vi "Turret_Execute.vi"() -> ()   [LabVIEW 2019]
uses:
  Turret_States.ctl
  <vilib>/Rock Robotics/WPI/ThirdParty/REV Robotics/SPARK MAX/Typedef/Spark MAX Control Type.ctl
  Globals/Turret_Globals.vi
  Globals/Sensor_Values.vi
panel:
  out "Waveform Chart":cluster{"Goal Wheel Position":dbl, dbl}(graph)
  in  "Kp_Degrees":dbl=0.07
  in  "Kd Aim":dbl=0.001
  in  "Ki Aim":dbl=1e-05
  in  "upper_limit(degrees)":dbl=135.0
  in  "lower_limit(degrees)":dbl=-83.0
  out "Turret_Spin_Speed":dbl
  in  "Kp Aim":dbl=0.06
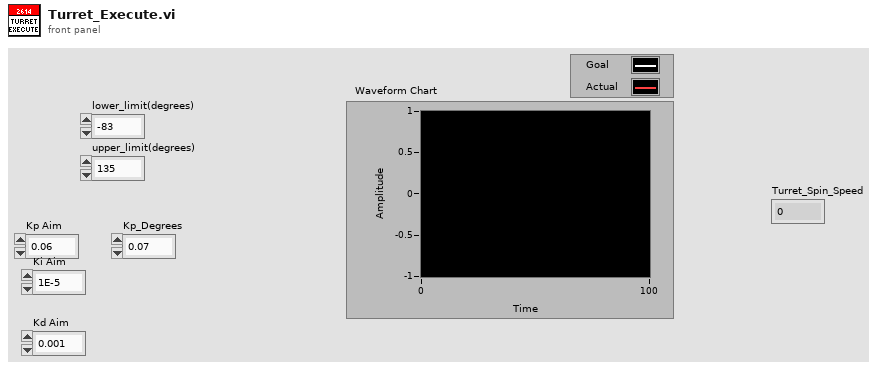
[diagram p1: front panel]
types:
  T1 = typedef "WPI_MotorControlDeviceRef.ctl" = cluster{"DeviceStatus":errorcluster, "Type":T2, "PWM":cluster{"PWM Channel":T3, "DeadBand":T4}, "CAN":cluster{"Device Number":u8, "SetOutput VI Ref":variant, "GetOutput VI Ref":variant, "Enable VI Ref":variant, "Disable VI Ref":variant, "Data":variant}, "Invert":bool, "DIO PWM":cluster{"PWM \"Enable\" Channel":T3, "DIOChannel":T5, "PWM Rate":dbl}}
  T2 = typedef "WPI_MotorControlType.ctl" = enum16{"PWM", "CAN", "DIO PWM"}
  T3 = typedef "FPGA_DIOPWMChannel.ctl" = enum8{"PWM 0", "PWM 1", "PWM 2", "PWM 3", "PWM 4", "PWM 5", "PWM 6", "PWM 7", "PWM 8", "PWM 9", "PWM MXP 0", "PWM MXP 1", "PWM MXP 2", "PWM MXP 3", "PWM MXP 4", "PWM MXP 5", "PWM MXP 6", "PWM MXP 7", "PWM MXP 8", "PWM MXP 9", "Invalid"}
  T4 = typedef "WPI_PWMDeadband.ctl" = cluster{"Name":string, "maxPositivePwm":i32, "minPositivePwm":i32, "centerPwm":i32, "maxNegativePwm":i32, "minNegativePwm":i32, "angularRange":u16}
  T5 = typedef "FPGA_DIOChannel.ctl" = enum8{"DIO 0", "DIO 1", "DIO 2", "DIO 3", "DIO 4", "DIO 5", "DIO 6", "DIO 7", "DIO 8", "DIO 9", "DIO MXP 0", "DIO MXP 1", "DIO MXP 2", "DIO MXP 3", "DIO MXP 4", "DIO MXP 5", "DIO MXP 6", "DIO MXP 7", "DIO MXP 8", "DIO MXP 9", "DIO MXP 10", "DIO MXP 11", "DIO MXP 12", "DIO MXP 13", "DIO MXP 14", "DIO MXP 15", "SPI Port CS1", "SPI Port CS2", "SPI Port CS3", "SPI Port MISO", "SPI Port MOSI", "Invalid"}
  T6 = typedef "Turret_States.ctl" = enum16{"Manual_Percent_Voltage", "Manual_Speed_Control", "Auto-Target", "Command_TurnToPosition", "Command_Auto_Target", "GoToZero"}
  T7 = typedef "Spark MAX Control Type.ctl" = enum16{"Percent VBus", "Voltage", "Velocity", "Position", "Smart Motion", "Current", "Smart Velocity"}
  T8 = typedef "Turret_Cluster.ctl" = cluster{"Auto-Target?":bool, "Control_State":T6, "Turret_Spin_Speed":dbl, "Turret_Spin_Speed_Control?":bool, "Step":dbl, "Parameter_1":dbl, "Parameter_2":dbl, "Parameter_3":dbl, "Auto_Notifier":refnum<notifier>, "GoToZero?":bool}
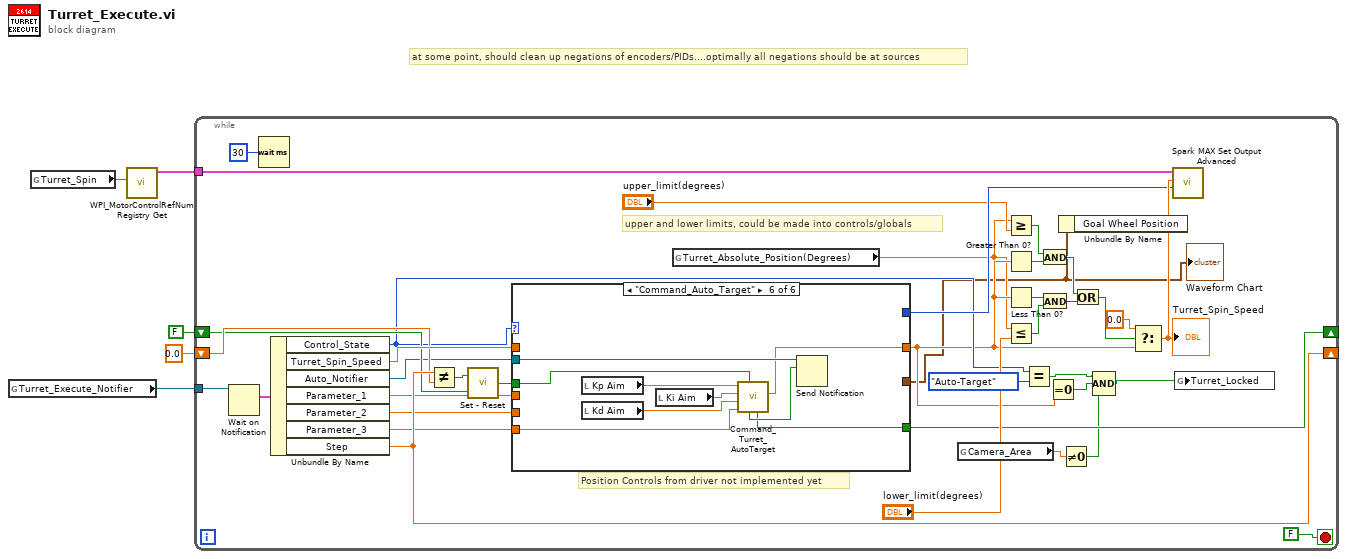
[diagram p0: block diagram]
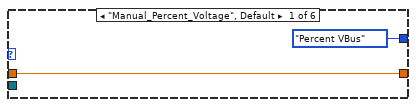
[diagram p2: hidden frame]
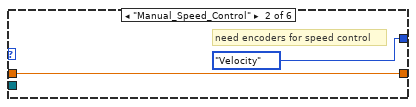
[diagram p3: hidden frame]
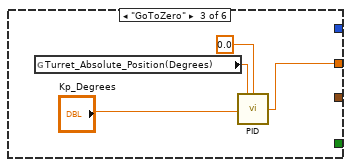
[diagram p4: hidden frame]
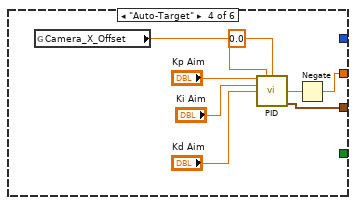
[diagram p5: hidden frame]
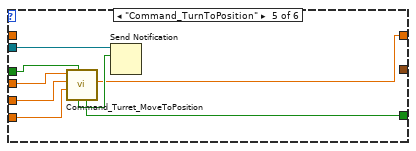
[diagram p6: hidden frame]
diagram:
  # "at some point, should clean up negations of encoders/PIDs....optimally all negations should be at sources"
  n1 = global read "Turret_Globals.vi" "Turret_Execute_Notifier"() -> (w5:refnum<notifier>)
  n2 = global read "Turret_Globals.vi" "Turret_Spin"() -> (w4:string)
  n3 = call <vilib>:"WPI_MotorControlRefNum Registry Get.vi"("refnum name"=w4) -> ("MotorControlDevRef"=w3:T1)  [unwired: 9 in, 1 out]
  n4 = while {
    tunnel: w5 -> [w42]
    tunnel: w3 -> [w32]
    shift-right: [w26] -> _
    shift-left: 0.0 ("Step") -> [w25]
    shift-right: [w17] -> _
    shift-left: FALSE ("Output") -> [w23]
    stop <- FALSE stop-if-true
    # "Position Controls from driver not implemented yet"
    # "upper and lower limits, could be made into controls/globals"
    n5 = Wait on Notification(notifier=w42) -> (notification=w41:T8)  [unwired: 3 in, 3 out]
    n6 = Wait (ms)(milliseconds to wait=u32 30) -> ()  [unwired: 1 out]
    n7 = Unbundle By Name(w41) -> ("Control_State"=w16:T6, "Turret_Spin_Speed"=w40:dbl, "Auto_Notifier"=w18:refnum<notifier>, "Parameter_1"=w22:dbl, "Parameter_2"=w21:dbl, "Parameter_3"=w20:dbl, "Step"=w26:dbl)
    n8 = Not Equal?(x=w26, y=w25) -> (x != y?=w24:bool)
    n9 = call "Set - Reset.vi"("Reset"=w23, "Set"=w24) -> ("Output"=w19:bool)
    n10 = case shown="\"Command_Auto_Target\"" w16 {
      tunnel: w40 -> [w45 w46 _ _ _ _]
      tunnel: [w45 w46 w48 w55 w60 w68] -> w14
      tunnel: [Spark_MAX_Control_Type."Percent VBus" ("Control Mode") Spark_MAX_Control_Type."Velocity" ("Control Mode") _ _ _ _] -> w30
      tunnel: w22 -> [_ _ _ _ w67 _]
      tunnel: w21 -> [_ _ _ _ w66 _]
      tunnel: w20 -> [_ _ _ _ w65 w73]
      tunnel: w19 -> [_ _ _ _ w64 w72]
      tunnel: w18 -> [_ _ _ _ w63 w71]
      tunnel: [_ _ _ _ w61 w69] -> w17
      tunnel: [_ _ _ w52 _ _] -> w7
      frame "Manual_Percent_Voltage", Default {
      }
      frame "Manual_Speed_Control" {
        # "need encoders for speed control"
      }
      frame "GoToZero" {
        n11 = global read "Sensor_Values.vi" "Turret_Absolute_Position(Degrees)"() -> (w51:dbl)
        n12 = call "PID.vi"("Kp"="Kp_Degrees", "Process Variable"=w51, "Goal"=0.0) -> ("Command"=w48:dbl)  [unwired: 10 in, 2 out]
      }
      frame "Auto-Target" {
        n13 = global read "Sensor_Values.vi" "Camera_X_Offset"() -> (w56:dbl)
        n14 = call "PID.vi"("Kp"="Kp Aim", "Process Variable"=w56, "Goal"=0.0, "Ki"="Ki Aim", "Kd"="Kd Aim") -> ("Command"=w58:dbl, "PID Tracking"=w52:cluster{"Goal Wheel Position":dbl, dbl})  [unwired: 8 in, 1 out]
        n15 = Negate(x=w58) -> (-x=w55:dbl)
      }
      frame "Command_TurnToPosition" {
        n16 = call "Command_Turret_MoveToPosition.vi"("Startup"=w64, "Timeout"=w65, "Speed"=w66, "Goal_Position"=w67) -> ("Turret_Speed"=w60:dbl, "Reint"=w61:bool, "Completed"=w62:bool)  [unwired: 5 in]
        n17 = Send Notification(notification=w62, notifier=w63) -> ()  [unwired: 1 in, 2 out]
      }
      frame "Command_Auto_Target" {
        n18 = local read "Kp Aim"() -> (w76:dbl)
        n19 = local read "Kd Aim"() -> (w74:dbl)
        n20 = local read "Ki Aim"() -> (w75:dbl)
        n21 = call "Command_Turret_AutoTarget.vi"("Startup"=w72, "Timeout"=w73, "Kd"=w74, "Ki"=w75, "Kp"=w76) -> ("Turret_Speed"=w68:dbl, "Reint"=w69:bool, "Completed"=w70:bool)  [unwired: 4 in]
        n22 = Send Notification(notification=w70, notifier=w71) -> ()  [unwired: 1 in, 2 out]
      }
    }
    "Waveform Chart" <- w7
    n23 = global read "Sensor_Values.vi" "Turret_Absolute_Position(Degrees)"() -> (w8:dbl)
    n24 = global read "Sensor_Values.vi" "Camera_Area"() -> (w10:dbl)
    n25 = Greater Or Equal?(x=w8, y="upper_limit(degrees)") -> (x >= y?=w39:bool)
    n26 = Greater Than 0?(x=w14) -> (x > 0?=w38:bool)
    n27 = Less Than 0?(x=w14) -> (x < 0?=w37:bool)
    n28 = Less Or Equal?(x=w8, y="lower_limit(degrees)") -> (x <= y?=w29:bool)
    n29 = Equal?(x=w16, y=Turret_States."Auto-Target") -> (x = y?=w12:bool)
    n30 = And(x=w39, y=w38) -> (x .and. y?=w35:bool)
    n31 = And(x=w37, y=w29) -> (x .and. y?=w36:bool)
    n32 = Equal To 0?(x=w14) -> (x = 0?=w11:bool)
    n33 = Unbundle By Name(w7) -> ()  [unwired: 1 out]
    n34 = Not Equal To 0?(x=w10) -> (x != 0?=w9:bool)
    n35 = Or(x=w35, y=w36) -> (x .or. y?=w6:bool)
    n36 = Compound Arithmetic op=AND(w12, w11, w9) -> (w13:bool)
    n37 = Select(t=0.0, s=w6, f=w14) -> (s? t:f=w31:dbl)
    "Turret_Spin_Speed" <- w31
    n38 = call <vilib>:"Spark MAX Set Output Advanced.vi"("Control Mode"=w30, "Setpoint"=w31, "MotorControlDevRef"=w32) -> ()  [unwired: 7 in, 2 out]
    n39 = global write "Turret_Globals.vi" "Turret_Locked"(w13) -> ()
  }
